vi "Preferences.vi"(7 "FileList":refnum<vi>, 11 "Files":T1[](array[typedef])) -> (0 "Settings out":T2={"Name of test"="", "Date"=timestamp(0 s since 1904-01-01), "Location"="", "Template"="", "Soundcard"="", "resolution"=32, "Sampling rate"=48000, "Ch1 Gain "=25.0, "Ch2 Gain"=10.0, "Sample time (s)"=0.3, "Pre-trigger (s)"=0.01, "Hammer Threshold"=10.0, "Positions"=12, "Taps/Position"=5, "Set Names"="", "Freq resolution"=10.0, "Hammer cutoff"=0.0, "Mic cutoff"=0.0, "Double bounce "=0.0, "Hammer Cal"=10.0, "dB Offset"=0.0, "Accel Cal"=10.0, "Vibrometer Cal"=0.0, "Mic Cal"=0.0, "Output"=2, "Voltage Cal"=0.01, "Vibrometer Port"="ASRL27::INSTR", "Range"=4, "High Pass"=2, "Bandwidth"=4, "X Range"=[], "Y Range"=[], "dB Spread"=0.0, "Trigger"=0, "Ch_1"=25, "Ch_2"=25, "flip?"=FALSE, "60Hz"=FALSE, "Time offset"=0.0, "Piezo Cal"=1.0, "Default Notes"=""} {"Ch_2" min=1 step=1; "Ch_1" min=1 max=100 step=1; "Trigger" items=["Hammer (force)", "Self-tap", "Spacebar"]; "Bandwidth" items=["1 kHz"=1, "5 kHz"=5, "10 kHz"=10, "25 kHz"=25, "50 kHz"=50, "100 kHz"=100]; "High Pass" items=["Off", "13 Hz", "104 Hz"]; "Range" items=["10 mm/s"=1, "20 mm/s"=2, "50 mm/s"=5, "100 mm/s"=10, "200 mm/s"=20, "500 mm/s"=50, "1 m/s"=100, "2 m/s"=200]; "Output" items=["Accelerometer", "Speed (from acceleration)", "Microphone", "Vibrometer", "Piezo"]; "Voltage Cal" format="%#_13g"; "Ch2 Gain" format="%#_13g"; "Ch1 Gain" format="%#_13g"; "Double bounce" min=0.0; "Mic cutoff" min=0.0 format="%#_4g"; "Hammer cutoff" min=0.0 format="%#_4g"; "Freq resolution" min=0.0; "Pre-trigger (s)" format="%#_13g"; "Date" format="%<%H:%M\n%d/%m/%y>T"; "resolution" items=["16 bit"=16, "24 bit"=24, "32 bit"=32]; "Sampling rate" items=["22050 samp/s"=22050, "44100 samp/s"=44100, "48000 samp/s"=48000]}, 1 "Success?":bool, 3 "Fixed Files":T1[](array[typedef]))   [LabVIEW 2022 SP3]
uses:
  PreferencesControl.ctl
  Curtin1_Label.ctl
  Mic/Mic_Global.vi
panel:
  out "Cover":bool
  in  "Tab Control":T3(tab)
  in  "CSV?":bool=TRUE
  in  "DAQ":bool
  in  "Vibrometer":bool
  in  "View":bool
  in  "Device":u16(ring) items=["BuerginBase Microphone", "MacBook Pro Microphone", "Reincubate", "Microsoft Teams Audio", "Jump Desktop Microphone", "Jump Desktop Audio", "ZoomAudioDevice"]
  out "Data Folder:":path=path "/Users/crogers/Desktop/Curtin2/Data"
  in  "Data Folder":bool
  out "Path to preferences":path
  out "Current ScratchPad Settings":string
  in  "Trigger":u16(ring) items=["Hammer (force)", "Self-tap"]
  in  "60Hz?":bool
  in  "Add Color":bool
  in  "Viewing":T4={"Alerts"=FALSE, "Log X Axis"=TRUE, "dB scale"=TRUE, "Averaging"=TRUE, "Fade"=0.8181818181818182, "Centroids?"=TRUE} {"Fade" scale=0.0..1.0}
  in  "Plot Colors":u16(ring) items=["Last Saved", "24 Colors"]
  in  "Note Files":u16(ring) items=["Default Notes", "Laser Notes", "Original Notes", "Testing Notes"]
  in  "Default Notes":string
  in  "Save As":bool
  in  "remove csv":bool
  in  "Reset":bool
  in  "Type":bool
  in  "Name":string(combo)
  in  "Selection":T5(radio)
  in  "open Folder":bool
  in  "Cancel Button":bool
  in  "OK Button":bool
  out "Version":string
  # "Hz"
  # "dB"
  # "dB"
  # "sec"
  # "sec"
  # "mV/Pa"
  # "mV/m/s2"
  # "mV/mm/s"
  # "V/N"
  # "sec"
  # "sec"
  # "mV/N"
  # "a.u."
  # "a.u."
  # "sec"
  # "not visible"
  # "no fade"
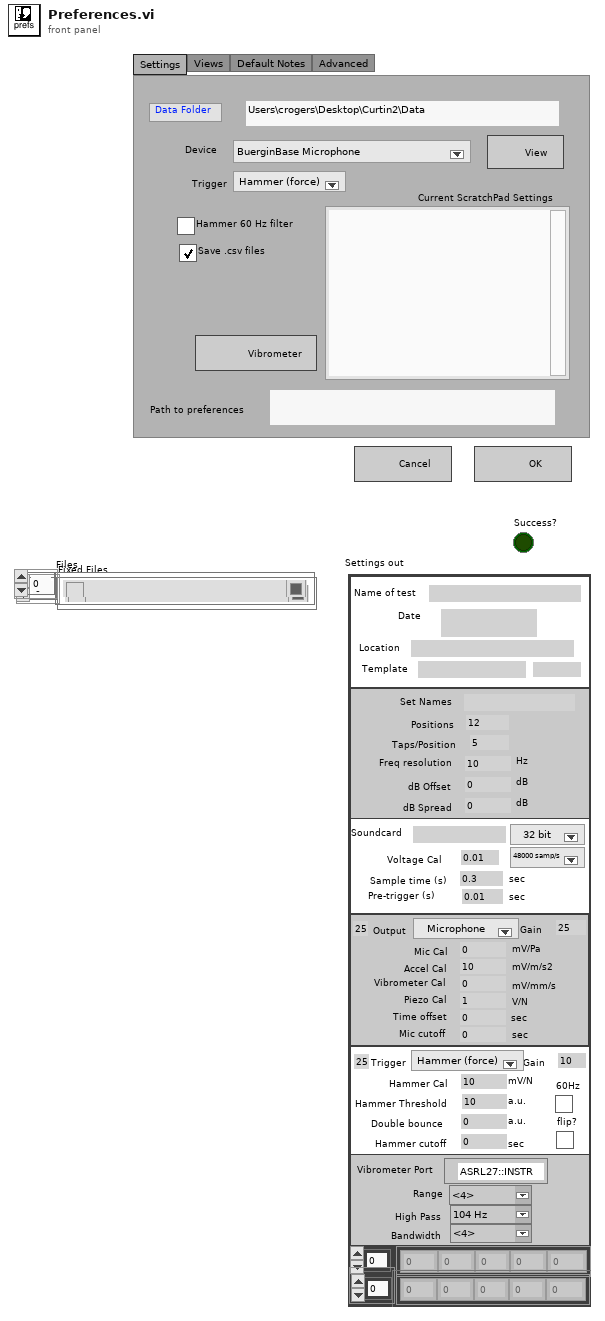
[diagram p1: front panel]
types:
  T1 = typedef "Curtin1_Label.ctl" = cluster{"Show?":bool, "Name":string, "Color":u32, "Path":path, "Show Notes":bool}
  T2 = typedef "PreferencesControl.ctl" = cluster{"Name of test":string, "Date":timestamp, "Location":string, "Template":string, "Soundcard":string, "resolution":u16, "Sampling rate":u16, "Ch1 Gain ":dbl, "Ch2 Gain":dbl, "Sample time (s)":dbl, "Pre-trigger (s)":dbl, "Hammer Threshold":dbl, "Positions":i16, "Taps/Position":i16, "Set Names":string, "Freq resolution":dbl, "Hammer cutoff":dbl, "Mic cutoff":dbl, "Double bounce ":dbl, "Hammer Cal":dbl, "dB Offset":dbl, "Accel Cal":dbl, "Vibrometer Cal":dbl, "Mic Cal":dbl, "Output":u16, "Voltage Cal":dbl, "Vibrometer Port":refnum<visa-resource-name>, "Range":u16, "High Pass":u16, "Bandwidth":u16, "X Range":cluster{"Minimum":dbl, "Maximum":dbl, "Increment":dbl, "Minor Increment":dbl, "Start":dbl}[], "Y Range":cluster{"Minimum":dbl, "Maximum":dbl, "Increment":dbl, "Minor Increment":dbl, "Start":dbl}[], "dB Spread":dbl, "Trigger":u16, "Ch_1":u8, "Ch_2":u8, "flip?":bool, "60Hz":bool, "Time offset":dbl, "Piezo Cal":dbl, "Default Notes":string}
  T3 = enum32{"Settings", "Views", "Default Notes", "Advanced"}
  T4 = cluster{"Alerts":bool, "Log X Axis":bool, "dB scale":bool, "Averaging":bool, "Fade":dbl, "Centroids?":bool}
  T5 = enum32{"No Selection", "Rename", "Recalculate", "Export", "Delete", "Duplicate"}
  T6 = enum32{"Invalid", "Default", "Floating", "Floating/Auto-Hide", "Modal"}
  T7 = enum16{"big-endian, network order", "native, host order", "little-endian"}
  T8 = enum32{"No Selection", "Rename", "Recalculate", "Export", "Delete"}
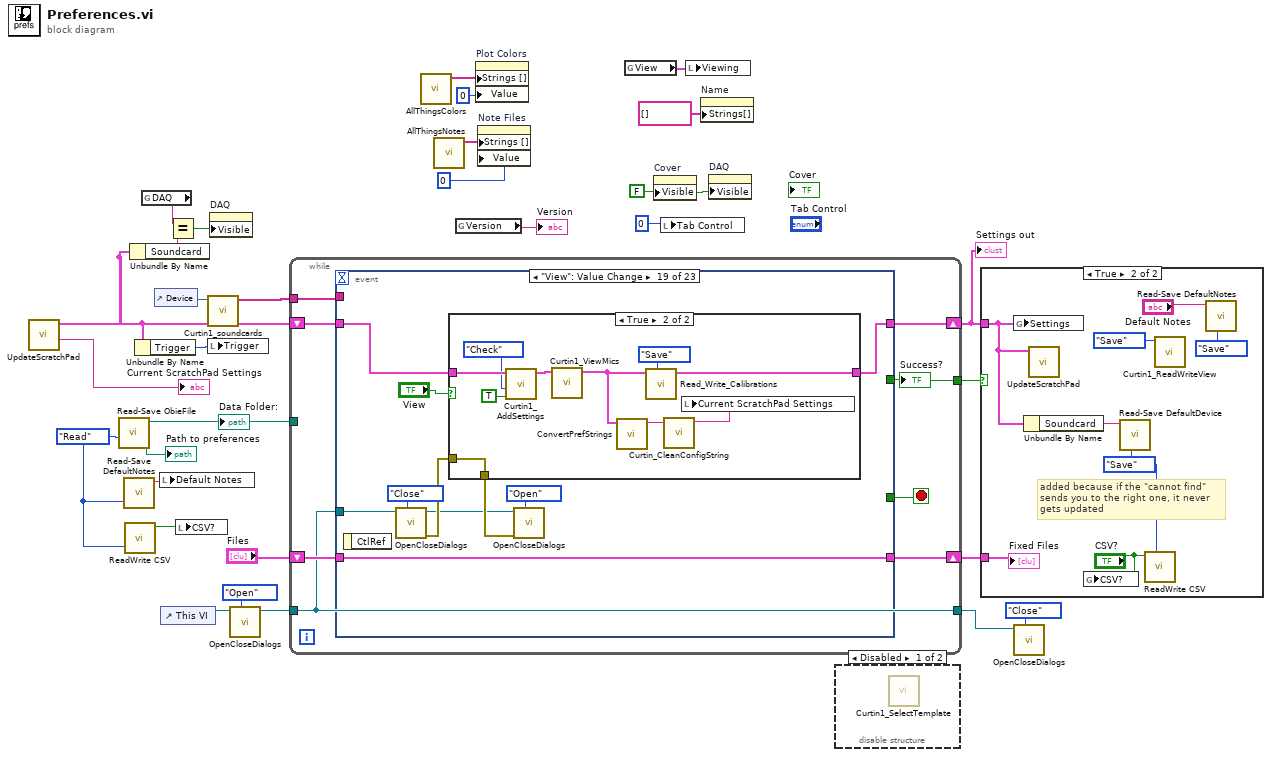
[diagram p0: block diagram]
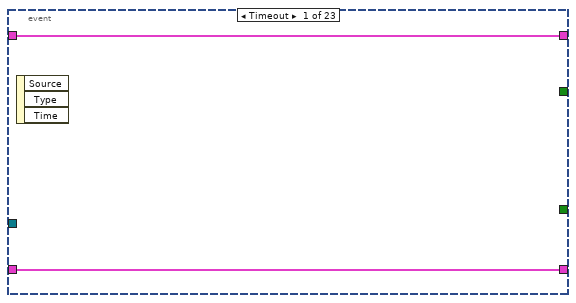
[diagram p4: hidden frame]
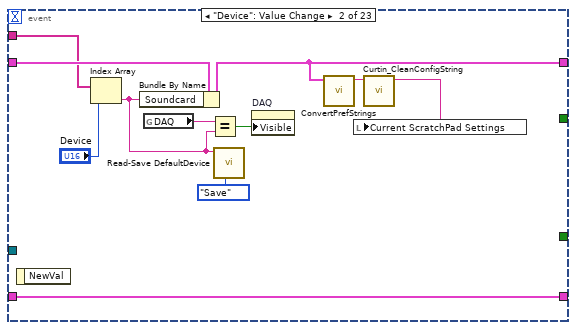
[diagram p5: hidden frame]
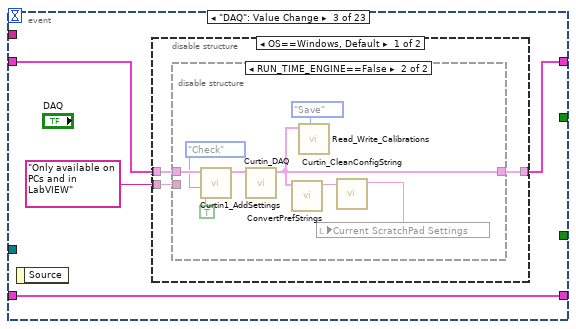
[diagram p6: hidden frame]
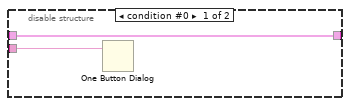
[diagram p7: hidden frame]
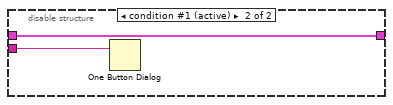
[diagram p8: hidden frame]
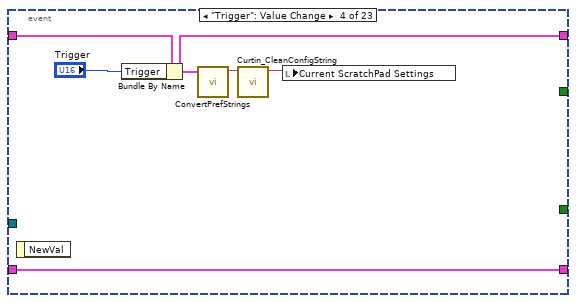
[diagram p9: hidden frame]
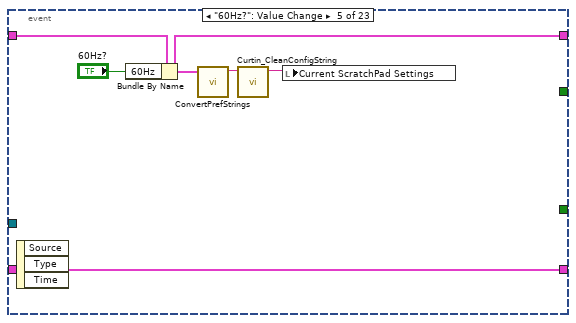
[diagram p10: hidden frame]
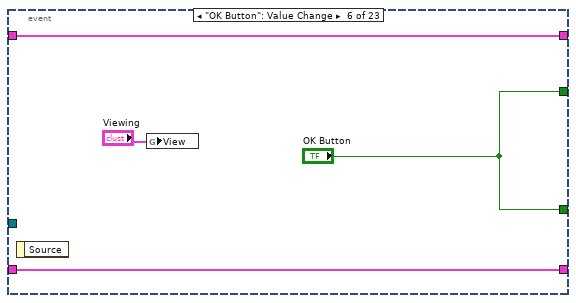
[diagram p11: hidden frame]
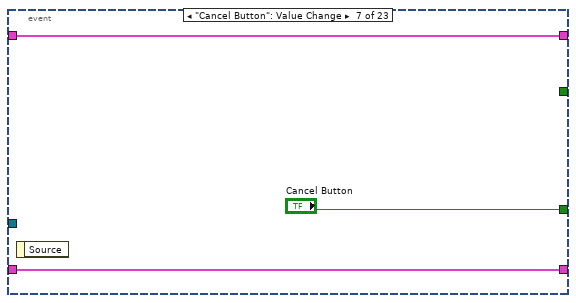
[diagram p12: hidden frame]
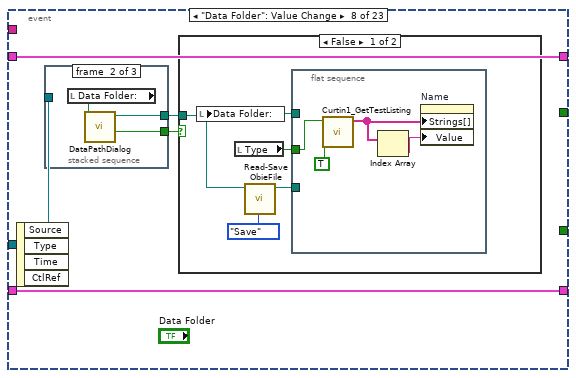
[diagram p13: hidden frame]
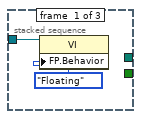
[diagram p14: hidden frame]
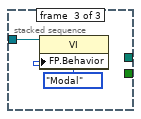
[diagram p15: hidden frame]
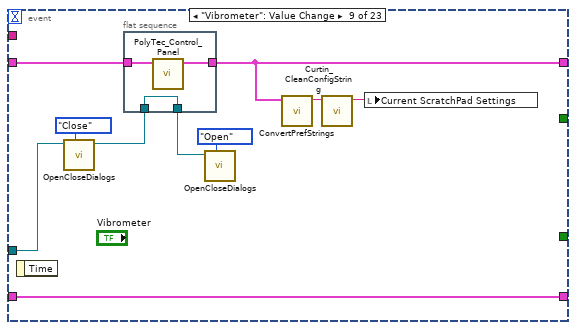
[diagram p17: hidden frame]
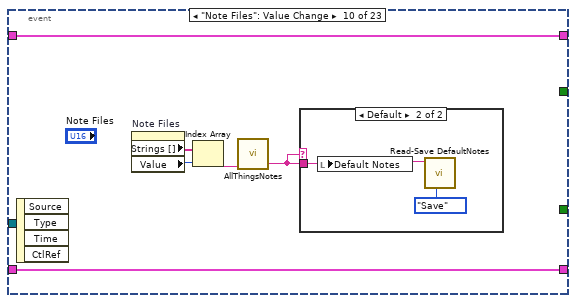
[diagram p18: hidden frame]
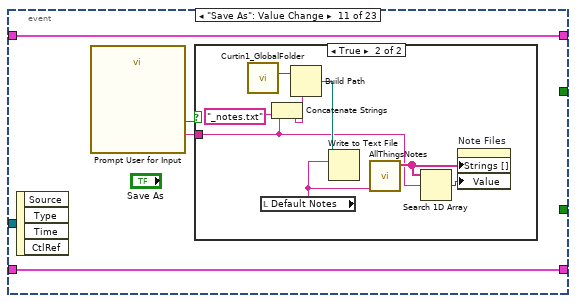
[diagram p20: hidden frame]
diagram:
  w10 = FALSE ("Visible")
  w2 = enum16{"Save", "Read"}."Read" ("Task")
  n1 = call "UpdateScratchPad.vi"() -> ("Settings"=→"Current ScratchPad Settings":string, "Settings Out"=w9:T2)  [unwired: 10 in]
  n2 = call "Read-Save ObieFile.vi"("Task"=w2) -> ("Pref Path"=→"Path to preferences":path, "DataPath Out"=w25:path)  [unwired: 8 in, 1 out]
  "Data Folder:" <- w25
  n3 = call "Read-Save DefaultNotes.vi"("Task"=w2) -> ("Notes Out"=w29:string)  [unwired: 9 in, 1 out]
  n4 = call "ReadWrite CSV.vi"("Task"=w2) -> ("csv Out"=w1:bool)  [unwired: 10 in]
  n5 = Unbundle By Name(w9) -> ("Soundcard"=w12:string)
  n6 = Unbundle By Name(w9) -> ("Trigger"=w20:u16)
  n7 = global read "Mic_Global.vi" "DAQ"() -> (w11:string)
  n8 = control-ref of="Device"() -> (w24:refnum<vi>)
  n9 = local write "Default Notes"(w29) -> ()
  n10 = control-ref of="This VI"() -> (w6:refnum<vi>)
  n11 = Equal?(x=w11, y=w12) -> (x = y?=w13:bool)
  n12 = local write "CSV?"(w1) -> ()
  n13 = call "Curtin1_soundcards.vi"("Settings In"=w9, "device:"=w24) -> ("Settings Out"=w19:T2, "Devices"=w26:string[])  [unwired: 8 in]
  n14 = local write "Trigger"(w20) -> ()
  n15 = property on="DAQ" class="Bool"("Visible"=w13) -> ()  [unwired: 2 in, 2 out]
  n16 = call "OpenCloseDialogs.vi"("Task"=enum16{"Open", "Close"}."Open", "VI in"=w6) -> ("VI out"=w3:refnum<vi>)  [unwired: 8 in, 1 out]
  n17 = while {
    tunnel: w26 -> [w39]
    shift-right: [w37] -> w30
    shift-left: w19 -> [w38]
    tunnel: [w36] -> w28
    tunnel: w25 -> [_]
    shift-right: [w35] -> w16
    shift-left: "Files" -> [w34]
    tunnel: [w33] -> w4
    tunnel: w3 -> [w33]
    stop <- w40 stop-if-true
    n18 = event shown="[18] \"View\": Value Change" {
      selector: _ -> [_ _ _ _ _ _ _ _ _ _ _ _ _ _ _ _ _ _ _ _ _ _ _]
      dyn-events: _ -> [_ _ _ _ _ _ _ _ _ _ _ _ _ _ _ _ _ _ _ _ _ _ _]
      timeout: _ -> [_ _ _ _ _ _ _ _ _ _ _ _ _ _ _ _ _ _ _ _ _ _ _]
      tunnel: [_ _ _ _ _ "OK Button" "Cancel Button" _ _ _ _ _ _ _ _ _ _ _ _ _ _ _ w245] -> w40
      tunnel: w39 -> [_ w51 _ _ _ _ _ _ _ _ _ _ _ _ _ _ _ _ _ _ _ _ _]
      tunnel: [_ _ _ _ _ "OK Button" _ _ _ _ _ _ _ _ _ _ _ _ _ _ _ _ _] -> w36
      tunnel: w38 -> [w42 w52 w54 w78 w84 w87 w90 w96 w120 w130 w136 w146 w153 w164 w169 w179 w185 w187 w196 w211 w221 w241 w244]
      tunnel: [w42 w44 w55 w74 w81 w87 w90 w96 w118 w130 w136 w146 w153 w164 w169 w179 w185 w187 w194 w211 w221 w241 w244] -> w37
      tunnel: [w41 w50 w57 w76 w83 w85 w89 w94 w121 w125 w133 w145 w147 w163 w168 w177 w184 w186 w195 w210 w220 w242 w243] -> w35
      tunnel: w34 -> [w41 w50 w57 w76 w83 w85 w89 w94 w121 w125 w133 w145 w147 w163 w168 w177 w184 w186 w195 _ w220 w242 w243]
      tunnel: w33 -> [_ _ _ _ _ _ _ w92 w115 _ _ _ _ _ _ _ _ _ w192 _ w217 _ _]
      event Timeout {
        n19 = event-data() -> ()  [unwired: 1 in, 3 out]
      }
      event "Device": Value Change {
        n20 = event-data() -> ()  [unwired: 1 in, 1 out]
        n21 = Index Array(array=w51, index="Device") -> (element=w46:string)
        n22 = Bundle By Name(cluster=w52, "Soundcard"=w46) -> (w44:T2)
        n23 = global read "Mic_Global.vi" "DAQ"() -> (w48:string)
        n24 = Equal?(x=w48, y=w46) -> (x = y?=w47:bool)
        n25 = call "Read-Save DefaultDevice.vi"("Task"=enum16{"Save", "Read"}."Save", "Soundcard"=w46) -> ()  [unwired: 8 in, 2 out]
        n26 = property on="DAQ" class="Bool"("Visible"=w47) -> ()  [unwired: 2 in, 2 out]
        n27 = call "ConvertPrefStrings.vi"("Settings"=w44) -> ("String Out"=w45:string)  [unwired: 9 in, 1 out]
        n28 = call "Curtin_CleanConfigString.vi"("String in"=w45) -> ("String out"=w43:string)  [unwired: 10 in]
        n29 = local write "Current ScratchPad Settings"(w43) -> ()
      }
      event "DAQ": Value Change {
        n30 = event-data() -> ()  [unwired: 1 in, 1 out]
        n31 = disable-structure shown="OS==Windows, Default" {
          disable-tunnel: "Only available on PCs and in LabVIEW" ("message") -> [w60 w72]
          disable-tunnel: w54 -> [w59 w71]
          disable-tunnel: [w58 w71] -> w55
          frame condition #0 {
            n32 = disable-structure shown="RUN_TIME_ENGINE==False" {
              disable-tunnel: w60 -> [w62 _]
              disable-tunnel: w59 -> [w61 w70]
              disable-tunnel: [w61 w68] -> w58
              frame condition #0 {
                n33 = One Button Dialog(message=w62) -> ()  [unwired: 1 in, 1 out]
              }
              frame condition #1 (active) {
                n34 = call "Curtin1_AddSettings.vi"("Date?"=TRUE, "Check?"=enum16{"Ignore", "Check", "Replace"}."Check", "Settings in"=w70) -> ("Settings Out"=w69:T2)  [unwired: 7 in, 1 out]
                n35 = call "Curtin_DAQ.vi"("Settings"=w69) -> ("Settings out"=w68:T2)  [unwired: 10 in]
                n36 = call "ConvertPrefStrings.vi"("Settings"=w68) -> ("String Out"=w66:string)  [unwired: 9 in, 1 out]
                n37 = call "Read_Write_Calibrations.vi"("Task"=enum16{"Save", "Read", "List"}."Save", "Settings in"=w68) -> ()  [unwired: 7 in, 3 out]
                n38 = call "Curtin_CleanConfigString.vi"("String in"=w66) -> ("String out"=w65:string)  [unwired: 10 in]
                n39 = local write "Current ScratchPad Settings"(w65) -> ()
              }
            }
          }
          frame condition #1 (active) {
            n40 = One Button Dialog(message=w72) -> ()  [unwired: 1 in, 1 out]
          }
        }
      }
      event "Trigger": Value Change {
        n41 = event-data() -> ()  [unwired: 1 in, 1 out]
        n42 = Bundle By Name(cluster=w78, "Trigger"="Trigger") -> (w74:T2)
        n43 = call "ConvertPrefStrings.vi"("Settings"=w74) -> ("String Out"=w75:string)  [unwired: 9 in, 1 out]
        n44 = call "Curtin_CleanConfigString.vi"("String in"=w75) -> ("String out"=w73:string)  [unwired: 10 in]
        n45 = local write "Current ScratchPad Settings"(w73) -> ()
      }
      event "60Hz?": Value Change {
        n46 = event-data() -> ()  [unwired: 1 in, 3 out]
        n47 = Bundle By Name(cluster=w84, "60Hz"="60Hz?") -> (w81:T2)
        n48 = call "ConvertPrefStrings.vi"("Settings"=w81) -> ("String Out"=w82:string)  [unwired: 9 in, 1 out]
        n49 = call "Curtin_CleanConfigString.vi"("String in"=w82) -> ("String out"=w80:string)  [unwired: 10 in]
        n50 = local write "Current ScratchPad Settings"(w80) -> ()
      }
      event "OK Button": Value Change {
        n51 = event-data() -> ()  [unwired: 1 in, 1 out]
        n52 = global write "Mic_Global.vi" "View"("Viewing") -> ()
      }
      event "Cancel Button": Value Change {
        n53 = event-data() -> ()  [unwired: 1 in, 1 out]
      }
      event "Data Folder": Value Change {
        n54 = event-data() -> ()  [unwired: 1 in, 4 out]
        n55 = stacked-sequence {
          tunnel: [_ w100 _] -> w95
          tunnel: [_ w99 _] -> w93
          tunnel: w92 -> [w98 _ w103]
          frame #0 {
            n56 = property class="VI"(reference=w98, "FP.Behavior"=T6."Floating" ("Front Panel Window:Behavior")) -> ()  [unwired: 1 in, 2 out]
          }
          frame #1 {
            n57 = local read "Data Folder:"() -> (w101:path)
            n58 = call "DataPathDialog.vi"("Path"=w101) -> ("canceled?"=w99:bool, "Path out"=w100:path)  [unwired: 9 in]
          }
          frame #2 {
            n59 = property class="VI"(reference=w103, "FP.Behavior"=T6."Modal" ("Front Panel Window:Behavior")) -> ()  [unwired: 1 in, 2 out]
          }
        }
        n60 = case shown="False" w93 {
          tunnel: w95 -> [w105 _]
          frame False {
            n61 = local write "Data Folder:"(w105) -> ()
            n62 = local read "Type"() -> (w107:bool)
            n63 = call "Read-Save ObieFile.vi"("Task"=enum16{"Save", "Read"}."Save", "DataPath"=w105) -> ("DataPath Out"=w104:path)  [unwired: 7 in, 2 out]
            n64 = flat-sequence {
              tunnel: w105 -> [_]
              tunnel: w107 -> [w109]
              tunnel: w104 -> [_]
              frame #0 {
                n65 = call "Curtin1_GetTestListing.vi"("Rebuild"=TRUE, "Type"=w109) -> ("Array"=w111:string[])  [unwired: 9 in]
                n66 = Index Array(array=w111) -> (element=w110:string)  [unwired: 1 in]
                n67 = property on="Name" class="CmbBox"("Strings[]"=w111, "Value"=w110) -> ()  [unwired: 2 in, 2 out]
              }
            }
          }
          frame True {
          }
        }
      }
      event "Vibrometer": Value Change {
        n68 = event-data() -> ()  [unwired: 1 in, 1 out]
        n69 = call "OpenCloseDialogs.vi"("Task"=enum16{"Open", "Close"}."Close", "VI in"=w115) -> ("VI out"=w113:refnum<vi>)  [unwired: 8 in, 1 out]
        n70 = flat-sequence {
          tunnel: w120 -> [w124]
          tunnel: [w123] -> w118
          tunnel: [w122] -> w114
          tunnel: w113 -> [w122]
          frame #0 {
            n71 = call "PolyTec_Control_Panel.vi"("Settings in"=w124) -> ("Settings Out"=w123:T2)  [unwired: 8 in, 2 out]
          }
        }
        n72 = call "OpenCloseDialogs.vi"("Task"=enum16{"Open", "Close"}."Open", "VI in"=w114) -> ()  [unwired: 8 in, 2 out]
        n73 = call "ConvertPrefStrings.vi"("Settings"=w118) -> ("String Out"=w119:string)  [unwired: 9 in, 1 out]
        n74 = call "Curtin_CleanConfigString.vi"("String in"=w119) -> ("String out"=w117:string)  [unwired: 10 in]
        n75 = local write "Current ScratchPad Settings"(w117) -> ()
      }
      event "Note Files": Value Change {
        n76 = event-data() -> ()  [unwired: 1 in, 4 out]
        n77 = property on="Note Files" class="Ring (strict)"() -> ("Strings []"=w129:string[], "Value"=w127:u16)  [unwired: 2 in, 2 out]
        n78 = Index Array(array=w129, index=w127) -> (element=w128:string)
        n79 = call "AllThingsNotes.vi"("Choice"=w128) -> ("Text"=w126:string)  [unwired: 9 in, 1 out]
        n80 = case shown="Default" w126 {
          tunnel: w126 -> [_ w131]
          frame "" {
          }
          frame Default {
            n81 = local write "Default Notes"(w131) -> ()
            n82 = call "Read-Save DefaultNotes.vi"("Task"=enum16{"Save", "Read"}."Save", "Notes"=w131) -> ()  [unwired: 8 in, 2 out]
          }
        }
      }
      event "Save As": Value Change {
        n83 = event-data() -> ()  [unwired: 1 in, 4 out]
        n84 = call "Prompt User for Input"() -> ("Filename"=w134:string, "OK"=w135:bool)  [unwired: 17 in, 1 out]
        n85 = case shown="True" w135 {
          tunnel: w134 -> [_ w137]
          frame False {
          }
          frame True {
            n86 = call "Curtin1_GlobalFolder.vi"() -> ("LabVIEW Data Path"=w143:path)  [unwired: 1 in, 1 out]
            n87 = local read "Default Notes"() -> (w141:string)
            n88 = Concatenate Strings(w137, "_notes.txt" ("pattern")) -> (w140:string)
            n89 = Build Path(base path=w143, name or relative path=w140) -> (appended path=w142:path)
            n90 = Write to Text File(file (use dialog)=w142, text=w141) -> ()  [unwired: 2 in, 3 out]
            n91 = call "AllThingsNotes.vi"("Choice"=w141) -> ("Array"=w138:string[])  [unwired: 9 in, 1 out]
            n92 = Search 1D Array(1D array=w138, element=w137) -> (index of element=w139:i32)  [unwired: 1 in]
            n93 = property on="Note Files" class="Ring (strict)"("Strings []"=w138, "Value"=w139) -> ()  [unwired: 2 in, 2 out]
          }
        }
      }
      event "Default Notes": Value Change {
        n94 = event-data() -> ()  [unwired: 1 in, 4 out]
      }
      event "Selection": Value Change {
        n95 = event-data() -> ()  [unwired: 1 in, 2 out]
        n96 = local read "Type"() -> (w148:bool)
        n97 = call "Curtin1_AdvancedPrefs.vi"("Type"=w148, "Selection"="Selection", "Instrument:Test Name"="Name") -> ("Selection out"=w150:T8, "message"=w149:string)  [unwired: 7 in]
        n98 = local write "Selection"(w150) -> ()
        n99 = case shown="Default" w149 {
          selector: w149 -> [_ w158]
          tunnel: w148 -> [_ w155]
          frame "" {
          }
          frame Default {
            n100 = One Button Dialog(message=w158) -> ()  [unwired: 1 in, 1 out]
            n101 = call "Curtin1_GetTestListing.vi"("Rebuild"=TRUE, "Type"=w155) -> ("Array"=w157:string[])  [unwired: 9 in]
            n102 = Index Array(array=w157) -> (element=w156:string)  [unwired: 1 in]
            n103 = property on="Name" class="CmbBox"("Strings[]"=w157, "Value"=w156) -> ()  [unwired: 2 in, 2 out]
          }
        }
      }
      event "Type": Value Change {
        n104 = event-data() -> ()  [unwired: 1 in, 2 out]
        n105 = property on="Cover" class="Bool (strict)"("Visible"=TRUE) -> ()  [unwired: 2 in, 2 out]
        n106 = call "Curtin1_GetTestListing.vi"("Rebuild"=FALSE, "Type"="Type") -> ("Array"=w167:string[])  [unwired: 9 in]
        n107 = Index Array(array=w167) -> (element=w166:string)  [unwired: 1 in]
        n108 = property on="Name" class="CmbBox"("Strings[]"=w167, "Value"=w166) -> (error out=w160:errorcluster)  [unwired: 2 in, 1 out]
        n109 = property on="Cover" class="Bool (strict)"(error in=w160, "Visible"=FALSE) -> ()  [unwired: 1 in, 2 out]
      }
      event "Tab Control": Value Change {
        n110 = event-data() -> ("NewVal"=w170:T3)  [unwired: 1 in]
        n111 = case shown="\"Advanced\"" w170 {
          frame "Settings", Default {
          }
          frame "Advanced" {
            n112 = property on="Name" class="CmbBox"() -> ("Strings[]"=w173:string[])  [unwired: 2 in, 2 out]
            n113 = Array Size(array=w173) -> (size(s)=w172:i32)
            n114 = case shown="0" w172 {
              tunnel: string[] ["Loading..."] ("Strings []") -> [_ w174]
              frame Default {
              }
              frame 0 {
                # "First Run"
                n115 = property on="Type" class="Bool (strict)"("Val(Sgnl)"=FALSE ("Value (Signaling)")) -> ()  [unwired: 2 in, 2 out]
                n116 = property on="Name" class="CmbBox"("Strings[]"=w174) -> ()  [unwired: 2 in, 2 out]
              }
            }
          }
        }
      }
      event "Reset": Value Change {
        n117 = event-data() -> ()  [unwired: 1 in, 1 out]
        n118 = call "Curtin1_GlobalFolder.vi"() -> ("LabVIEW Data Path"=w176:path)  [unwired: 1 in, 1 out]
        n119 = call "DefaultSettings.vi"("Task"=enum16{"Load to VI", "Save to Disk"}."Save to Disk", "path (use dialog)"=w176) -> ("No Errors?"=w178:bool)  [unwired: 9 in]
        n120 = case shown="False" w178 {
          frame False {
            n121 = One Button Dialog(message="Error in saving files") -> ()  [unwired: 1 in, 1 out]
          }
          frame True {
            n122 = One Button Dialog(message="Success") -> ()  [unwired: 1 in, 1 out]
          }
        }
      }
      event "open Folder": Value Change {
        n123 = event-data() -> ()  [unwired: 1 in, 1 out]
        n124 = call "Curtin1_GlobalFolder.vi"() -> ("LabVIEW Data Path"=w183:path)  [unwired: 1 in, 1 out]
        n125 = call "OpenFolder.vi"("LabVIEW Data Path"=w183) -> ()  [unwired: 11 in]
      }
      event "Name": Value Change {
        n126 = event-data() -> ()  [unwired: 1 in, 4 out]
      }
      event "View": Value Change {
        n127 = event-data() -> ()  [unwired: 1 in, 1 out]
        n128 = call "OpenCloseDialogs.vi"("Task"=enum16{"Open", "Close"}."Close", "VI in"=w192) -> ("error out"=w189:errorcluster, "VI out"=w188:refnum<vi>)  [unwired: 8 in]
        n129 = case shown="True" "View" {
          tunnel: w196 -> [w199 w207]
          tunnel: [w199 w201] -> w194
          tunnel: [w198 w200] -> w190
          tunnel: w189 -> [w198 w200]
          frame False {
          }
          frame True {
            n130 = call "Curtin1_AddSettings.vi"("Date?"=TRUE, "Check?"=enum16{"Ignore", "Check", "Replace"}."Check", "Settings in"=w207) -> ("Settings Out"=w208:T2)  [unwired: 7 in, 1 out]
            n131 = call "Curtin1_ViewMics.vi"("Settings"=w208) -> ("Settings Out"=w201:T2)  [unwired: 10 in]
            n132 = call "ConvertPrefStrings.vi"("Settings"=w201) -> ("String Out"=w206:string)  [unwired: 9 in, 1 out]
            n133 = call "Read_Write_Calibrations.vi"("Task"=enum16{"Save", "Read", "List"}."Save", "Settings in"=w201) -> ()  [unwired: 7 in, 3 out]
            n134 = call "Curtin_CleanConfigString.vi"("String in"=w206) -> ("String out"=w205:string)  [unwired: 10 in]
            n135 = local write "Current ScratchPad Settings"(w205) -> ()
          }
        }
        n136 = call "OpenCloseDialogs.vi"("Task"=enum16{"Open", "Close"}."Open", "error in (no error)"=w190, "VI in"=w188) -> ()  [unwired: 7 in, 2 out]
      }
      event "Plot Colors": Value Change {
        n137 = event-data() -> ()  [unwired: 1 in, 1 out]
        n138 = flat-sequence {
          tunnel: "FileList" -> [w216]
          tunnel: [w215] -> w210
          frame #0 {
            # "load into CurrentColors"
            n139 = property on="Plot Colors" class="Ring (strict)"() -> ("Strings []"=w213:string[], "Value"=w214:u16)  [unwired: 2 in, 2 out]
            n140 = Index Array(array=w213, index=w214) -> (element=w212:string)
            n141 = call "AllThingsColors.vi"("Choice"=w212) -> ()  [unwired: 10 in, 1 out]
          }
          frame #1 {
            # "replot"
            n142 = call "Recolor.vi"("Array in"=w216) -> ("Files"=w215:T1[])  [unwired: 10 in]
          }
        }
      }
      event "Add Color": Value Change {
        n143 = event-data() -> ()  [unwired: 1 in, 1 out]
        n144 = stacked-sequence {
          tunnel: [_ w225 _] -> w219
          tunnel: [_ w224 _] -> w218
          tunnel: w217 -> [w222 _ w226]
          frame #0 {
            n145 = property class="VI"(reference=w222, "FP.Behavior"=T6."Floating" ("Front Panel Window:Behavior")) -> ()  [unwired: 1 in, 2 out]
          }
          frame #1 {
            n146 = call "Curtin_SaveColor.vi"() -> ("New Color"=w225:string, "Good?"=w224:bool)  [unwired: 10 in]
          }
          frame #2 {
            n147 = property class="VI"(reference=w226, "FP.Behavior"=T6."Modal" ("Front Panel Window:Behavior")) -> ()  [unwired: 1 in, 2 out]
          }
        }
        n148 = case shown="True" w218 {
          tunnel: w220 -> [_ w235]
          tunnel: w219 -> [_ w230]
          frame False {
          }
          frame True {
            # "Save color file"
            n149 = for {
              tunnel: w235 -> [w240] mode=indexing
              tunnel: [w239] -> w232 mode=indexing
              n150 = Unbundle By Name(w240) -> ("Color"=w239:u32)
            }
            n151 = call "GetColorFilePath.vi"("String"=w230) -> ("name"=w228:string, "path"=w229:path)  [unwired: 9 in]
            n152 = Write to Binary File(file (use dialog)=w229, data=w232, 5:FALSE ("prepend array or string size? (T)"), 9:T7."big-endian, network order" ("byte order (0:big-endian, network order)")) -> (error out=w231:errorcluster)  [unwired: 2 in, 2 out]
            n153 = case shown="No Error" w231 {
              tunnel: w228 -> [w237 _]
              frame No Error {
                n154 = call "AllThingsColors.vi"() -> ("Possible Colors"=w238:string[])  [unwired: 11 in]
                n155 = Search 1D Array(1D array=w238, element=w237) -> (index of element=w236:i32)  [unwired: 1 in]
                n156 = property on="Plot Colors" class="Ring (strict)"("Strings []"=w238, "Value"=w236) -> ()  [unwired: 2 in, 2 out]
              }
              frame Error {
              }
            }
          }
        }
      }
      event "remove csv": Value Change {
        n157 = event-data() -> ()  [unwired: 1 in, 1 out]
        n158 = call "Delete csv.vi"() -> ()  [unwired: 12 in]
      }
      event Panel Close? {
        w245 = TRUE ("Discard?")
        n159 = event-data() -> ()  [unwired: 1 in, 4 out]
        n160 = event-data("Discard?"=w245) -> ()  [unwired: 1 in, 1 out]
      }
    }
    "Success?" <- w36
  }
  "Settings out" <- w30
  n161 = call "AllThingsColors.vi"() -> ("Possible Colors"=w15:string[])  [unwired: 11 in]
  n162 = call "AllThingsNotes.vi"() -> ("Array"=w23:string[])  [unwired: 10 in, 1 out]
  n163 = global read "Mic_Global.vi" "Version"() -> (→"Version":string)
  n164 = property on="Plot Colors" class="Ring (strict)"("Strings []"=w15, "Value"=0) -> ()  [unwired: 2 in, 2 out]
  n165 = property on="Note Files" class="Ring (strict)"("Strings []"=w23, "Value"=0) -> ()  [unwired: 2 in, 2 out]
  n166 = global read "Mic_Global.vi" "View"() -> (w21:T4)
  n167 = property on="Cover" class="Bool (strict)"("Visible"=w10) -> ()  [unwired: 2 in, 2 out]
  n168 = local write "Tab Control"(0) -> ()
  n169 = local write "Viewing"(w21) -> ()
  n170 = property on="Name" class="CmbBox"("Strings[]"=string[] [] ("Strings []")) -> ()  [unwired: 2 in, 2 out]
  n171 = property on="DAQ" class="Bool"("Visible"=w10) -> ()  [unwired: 2 in, 2 out]
  n172 = disable-structure shown="Disabled" {
    frame Disabled {
      n173 = call "Curtin1_SelectTemplate.vi"() -> ()  [unwired: 10 in, 2 out]
    }
    frame Enabled {
    }
  }
  n174 = case shown="True" w28 {
    tunnel: w30 -> [_ w249]
    tunnel: w16 -> [_ w250]
    frame False {
    }
    frame True {
      w247 = enum16{"Save", "Read"}."Save" ("Task")
      # "added because if the \"cannot find\"\nsends you to the right one, it never\ngets updated"
      n175 = global write "Mic_Global.vi" "Settings"(w249) -> ()
      n176 = Unbundle By Name(w249) -> ("Soundcard"=w248:string)
      n177 = call "UpdateScratchPad.vi"("Settings"=w249) -> ()  [unwired: 9 in, 2 out]
      n178 = global write "Mic_Global.vi" "CSV?"("CSV?") -> ()
      n179 = call "Read-Save DefaultDevice.vi"("Task"=w247, "Soundcard"=w248) -> ()  [unwired: 8 in, 2 out]
      n180 = call "ReadWrite CSV.vi"("Task"=w247, "csv?"="CSV?") -> ()  [unwired: 9 in, 1 out]
      n181 = call "Curtin1_ReadWriteView.vi"("Task"=enum16{"Read", "Save"}."Save") -> ()  [unwired: 8 in, 3 out]
      n182 = call "Read-Save DefaultNotes.vi"("Task"=enum16{"Save", "Read"}."Save", "Notes"="Default Notes") -> ()  [unwired: 8 in, 2 out]
      "Fixed Files" <- w250
    }
  }
  n183 = call "OpenCloseDialogs.vi"("Task"=enum16{"Open", "Close"}."Close", "VI in"=w4) -> ()  [unwired: 8 in, 2 out]
